vi "getCurrentScanNumber.vi"(8 "error in (no error)":errorcluster) -> (0 "error out":errorcluster, 2 "block":i64, 3 "sample":i64)   [LabVIEW 2015, in "ESLSCDLL.lvlib"]
uses:
  ESLSCDLL.lvlib
  Globals.vi
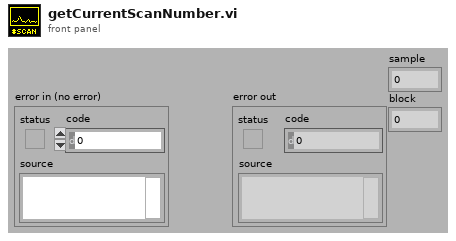
[diagram p1: front panel]
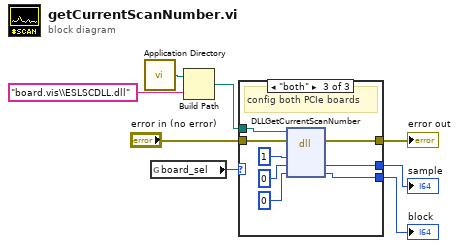
[diagram p0: block diagram]
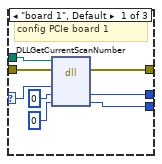
[diagram p2: hidden frame]
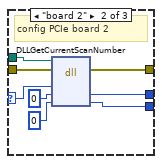
[diagram p3: hidden frame]
diagram:
  n1 = call <vilib>:"Application Directory.vi"() -> ("Application Directory"=w6:path)
  n2 = global read "Globals.vi" "board_sel"() -> (w7:enum32{"0", "board 1", "board 2", "both"})
  n3 = Build Path(base path=w6, name or relative path="board.vis\\ESLSCDLL.dll") -> (appended path=w4:path)
  n4 = case shown="\"both\"" w7 {
    selector: w7 -> [w16 w23 _]
    tunnel: "error in (no error)" -> [w15 w21 w30]
    tunnel: [w14 w20 w29] -> w1
    tunnel: w4 -> [w13 w22 w31]
    tunnel: [w12 w19 w26] -> w3
    tunnel: [w11 w18 w25] -> w2
    frame "board 1", Default {
      # "config PCIe board 1"
      n5 = dll-call lib="C:/Users/flori/Nextcloud/Dokumente/Stresing/Windows/lv64/board.vis/ESLSCDLL.dll" fn="DLLGetCurrentScanNumber" ("lwlscdll.dll:DLLWriteLongS0")(path in=w13, error in=w15, "drv"=w16, "sample"=i64 0, "block"=i64 0) -> (error out=w14:errorcluster, "sample"=w12:i64, "block"=w11:i64)  [unwired: 3 in, 1 out]
    }
    frame "board 2" {
      # "config PCIe board 2"
      n6 = dll-call lib="C:/Users/flori/Nextcloud/Dokumente/Stresing/Windows/lv64/board.vis/ESLSCDLL.dll" fn="DLLGetCurrentScanNumber" ("lwlscdll.dll:DLLWriteLongS0")(path in=w22, error in=w21, "drv"=w23, "sample"=i64 0, "block"=i64 0) -> (error out=w20:errorcluster, "sample"=w19:i64, "block"=w18:i64)  [unwired: 3 in, 1 out]
    }
    frame "both" {
      # "config both PCIe boards"
      n7 = dll-call lib="C:/Users/flori/Nextcloud/Dokumente/Stresing/Windows/lv64/board.vis/ESLSCDLL.dll" fn="DLLGetCurrentScanNumber" ("lwlscdll.dll:DLLWriteLongS0")(path in=w31, error in=w30, "drv"=u32 1, "sample"=i64 0, "block"=i64 0) -> (error out=w29:errorcluster, "sample"=w26:i64, "block"=w25:i64)  [unwired: 3 in, 1 out]
    }
  }
  "error out" <- w1
  "sample" <- w3
  "block" <- w2
